vi "Demo.vi"() -> ()   [LabVIEW 2021, in "Autocomplete popup.lvlib"]
uses:
  Autocomplete popup.lvlib
  subvis/input options.ctl
  <vilib>/Utility/miscctls.llb/LVPointTypeDef.ctl
panel:
  out "Accept?":bool
  out "String":string
  in  "OK Button":bool
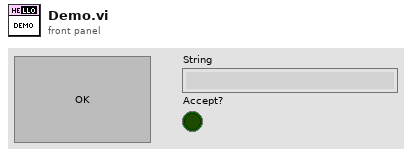
[diagram p1: front panel]
types:
  T1 = typedef "Autocomplete popup.lvlib/input options.ctl" = cluster{"Screen Coordinates":T2, "Width":u32, "max rows":i32, "List":string[], "init value":string}
  T2 = typedef "LVPointTypeDef.ctl" = cluster{"Horizontal":i16, "Vertical":i16}
  T3 = typedef "LVPositionTypeDef.ctl" = cluster{"Left":i32, "Top":i32}
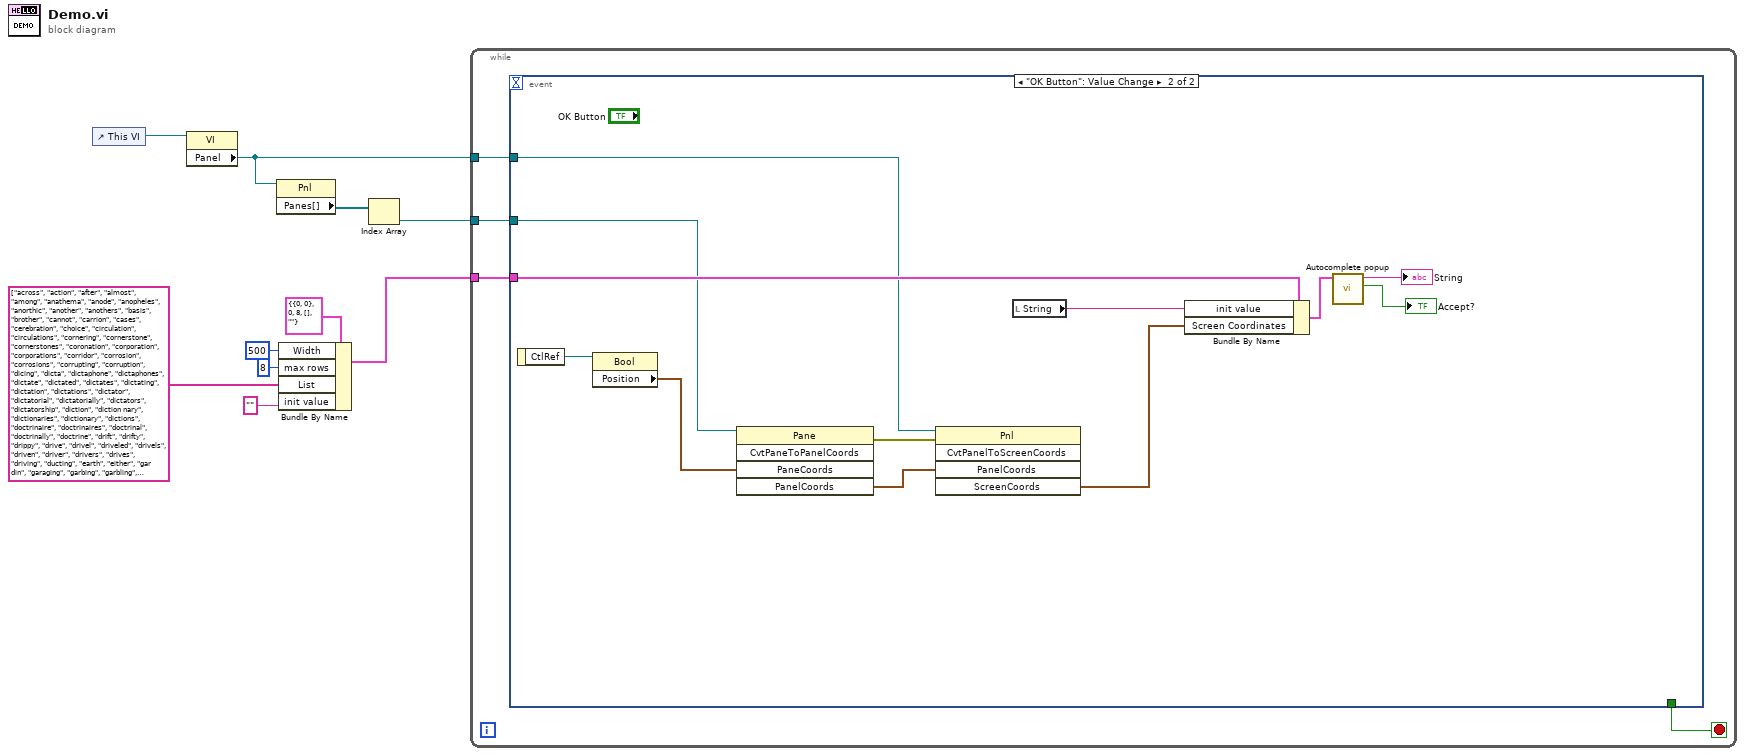
[diagram p0: block diagram]
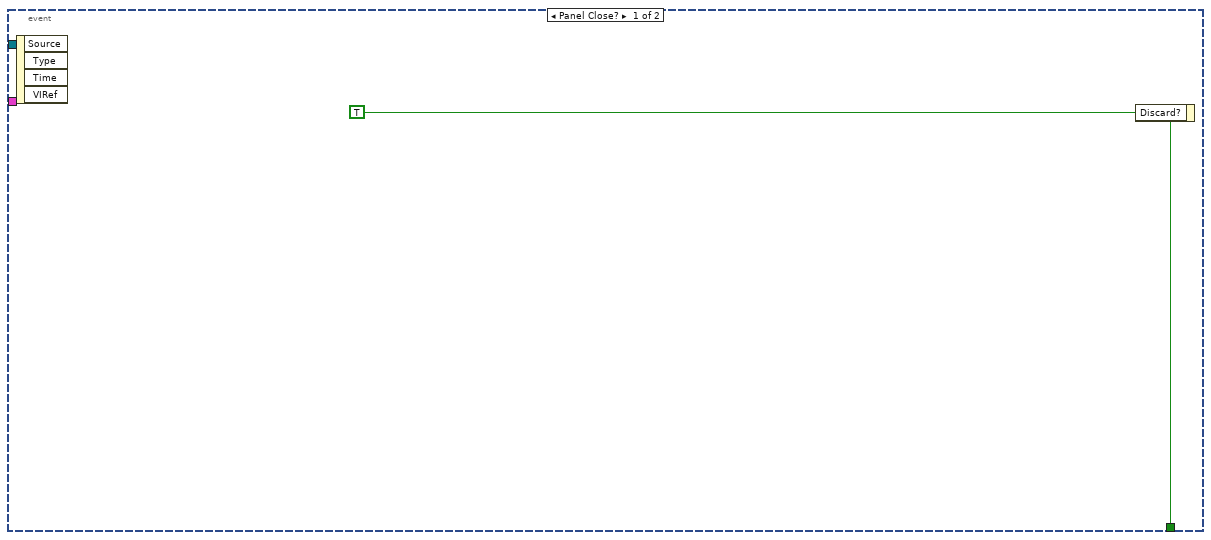
[diagram p2: hidden frame]
diagram:
  n1 = control-ref of="This VI"() -> (w5:refnum<vi>)
  n2 = property class="VI"(reference=w5) -> ("Panel"=w4:refnum<vi>)  [unwired: 1 in, 2 out]
  n3 = property class="Pnl"(reference=w4) -> ("Panes[]"=w3:refnum<vi>[])  [unwired: 1 in, 2 out]
  n4 = Bundle By Name(cluster=T1 {"Screen Coordinates"={"Horizontal"=0, "Vertical"=0}, "Width"=0, "max rows"=8, "List"=[], "init value"=""} ("input"), "Width"=u32 500, "max rows"=8, "List"=string[] ["across", "action", "after", "almost", "among", "anathema", "anode", "anopheles", "anorthic", "another", "anothers", "basis", "brother", "cannot", "carrion", "cases", "cerebration", "choice", "circulation", "circulations", "cornering", "cornerstone", "cornerstones", "coronation", "corporation", "corporations", "corridor", "corrosion", "corrosions", "corrupting", "corruption", "dicing", "dicta", "dictaphone", "dictaphones", "dictate", "dictated", "dictates", "dictating", "dictation", "dictations", "dictator", "dictatorial", "dictatorially", "dictators", "dictatorship", "diction", "diction nary", "dictionaries", "dictionary", "dictions", "doctrinaire", "doctrinaires", "doctrinal", "doctrinally", "doctrine", "drift", "drifty", "drippy", "drive", "drivel", "driveled", "drivels", "driven", "driver", "drivers", "drives", "driving", "ducting", "earth", "either", "gar din", "garaging", "garbing", "garbling", "garcon", "garde", "garden", "gardened", "gardener", "gardenia", "gardens", "gardner", "gargling", "goring", "habeas", "habited", "habits", "hebetate", "helicon", "helicopter", "helicopters", "heliotrope", "heliotropes", "heliotropism", "heliport", "hellcat", "hellcats", "hello", "helot", "helotries", "helotry", "helots", "hobbies", "hobbit", "hobbits", "hobblers", "hobbles", "hobbs", "hoboes", "hobos", "holdover", "hothead", "hotline", "hotlines", "hotpoint", "jasmine", "jasmines", "jason", "jaspers", "jests", "km art", "lateen", "lateens", "later", "lateral", "laterals", "lathe", "lather", "lathered", "latherer", "lathers", "lathery", "latter", "latterday", "latterly", "lattices", "leg ht", "legate", "legated", "legatee", "legates", "legato", "legator", "legatos", "leggett", "leghorn", "legit", "letter", "letters", "letterset", "lettersets", "liege", "lieges", "light", "likely", "lines", "lionize", "looking", "lottos", "machete", "machetes", "machine", "machined", "machines", "machinist", "machinists", "mahjong", "mahjongg", "mahoganies", "mahogany", "mahout", "mahouts", "majolica", "major", "majordomo", "majordomos", "majored", "majorette", "majorettes", "majoring", "majorities", "majority", "majors", "manta", "march", "massif", "mastic", "matador", "matadors", "matrimonial", "matrimonially", "matter", "matters", "matzo", "meant", "meccano", "mechanic", "mechanical", "mechanics", "mechanism", "mechanisms", "mechanist", "mechanistic", "mechanistically", "mechanists", "mechanize", "mechanized", "mechanizes", "meteor", "meter", "micas", "micatin", "michael", "michel", "michele", "michelin", "michelle", "michigan", "mickey", "microbic", "micron", "micronuclei", "microsoft", "might", "mighty", "mikes", "million", "mints", "minty", "mocha", "mochas", "mohair", "mohican", "mojave", "monday", "money", "monitor", "monster", "montage", "montana", "monte", "month", "monthly", "months", "monty", "mosaic", "mosaics", "moses", "mossback", "mossier", "mossiest", "mossing", "mosslike", "mossy", "mosts", "mother", "muses", "music", "musical", "musicale", "musicales", "musically", "musicals", "musician", "musicians", "mussily", "mussing", "mussy", "musts", "na iv", "na too", "naiad", "naifs", "nails", "naive", "naively", "naiveness", "naives", "naivete", "naivetes", "naivety", "natatorium", "nation", "national", "nationalism", "nationalist", "nationalistic", "nationalists", "nationalities", "nationality", "nationalize", "nationalizing", "nationally", "nationals", "nations", "neither", "nether", "nether land", "netherlander", "netherlanders", "netherlands", "netherworld", "netherworlds", "netter", "newark", "newborn", "newborns", "newer", "newly", "newmarket", "newport", "newsier", "newsy", "newton", "nicene", "niche", "niched", "niches", "niching", "nicknack", "nicknacks", "night", "nikes", "nikon", "nikons", "nohow", "notepad", "notes", "nothing", "notional", "noway", "palpitation", "palpitations", "parts", "person", "persons", "police", "policed", "polices", "policies", "policy", "poling", "polio", "polish", "polite", "politer", "politest", "politic", "politician", "politicians", "politicizing", "politick", "politicking", "politico", "politicos", "politics", "polities", "polity", "quickly", "reason", "reasons", "right", "rights", "sanative", "schedule", "scheduled", "scheduler", "schedulers", "schedules", "scheduling", "schema", "scheme", "scherzi", "scherzo", "schlep", "schlock", "schneider", "schnook", "schnooks", "scholar", "scholars", "scholl", "school", "schooled", "schooler", "schools", "schooner", "section", "semester", "semite", "senate", "senates", "senator", "senna", "sensate", "sentence", "sentenced", "sentences", "sentries", "she'd", "short", "sight", "situation", "sonant", "stuff", "swaged", "swayed", "swede", "swede en", "sweden", "swedes", "sweeper", "sweet", "sweeten", "sweetened", "sweetener", "sweeteners", "sweetening", "sweetens", "sweeter", "sweetie", "system", "systematic", "systematical", "systematics", "systematize", "systemic", "systemics", "systemize", "systemized", "systemizes", "systemizing", "systemless", "systems", "taurine", "taurines", "tautest", "technical", "touchiest", "toughest", "toughies", "touraine", "toured", "tourism", "tourist", "touristic", "touristically", "tourists", "tourneys", "until", "wander", "wanders", "wiggle", "wiggly", "wight", "wights", "winder", "winders", "windier", "winterkill", "wonder", "wonder full", "wondered", "wonderer", "wonderful", "wonderfully", "wonderfulness", "wonders", "wondrously"] ("words"), "init value"="") -> (w7:T1)
  n5 = Index Array(array=w3) -> (element=w2:refnum<vi>)  [unwired: 1 in]
  n6 = while {
    tunnel: w7 -> [w13]
    tunnel: w4 -> [w12]
    tunnel: w2 -> [w11]
    stop <- w14 stop-if-true
    n7 = event shown="[1] \"OK Button\": Value Change" {
      selector: _ -> [_ _]
      dyn-events: _ -> [_ _]
      timeout: _ -> [_ _]
      tunnel: [w15 _] -> w14
      tunnel: w13 -> [_ w25]
      tunnel: w12 -> [_ w20]
      tunnel: w11 -> [_ w19]
      event Panel Close? {
        w15 = TRUE ("Discard?")
        n8 = event-data() -> ()  [unwired: 1 in, 4 out]
        n9 = event-data("Discard?"=w15) -> ()  [unwired: 1 in, 1 out]
      }
      event "OK Button": Value Change {
        n10 = event-data() -> ("CtlRef"=w18:refnum<vi>)  [unwired: 1 in]
        n11 = property class="Bool"(reference=w18) -> ("Position"=w17:T3)  [unwired: 1 in, 2 out]
        n12 = invoke class="Pane" method="CvtPaneToPanelCoords"(reference=w19, "PaneCoords"=w17) -> (error out=w22:errorcluster, "PanelCoords"=w21:T2)  [unwired: 3 in, 3 out]
        n13 = invoke class="Pnl" method="CvtPanelToScreenCoords"(reference=w20, error in=w22, "PanelCoords"=w21) -> ("ScreenCoords"=w16:T2)  [unwired: 2 in, 4 out]
        n14 = local read "String"() -> (w24:string)
        n15 = Bundle By Name(cluster=w25, "init value"=w24, "Screen Coordinates"=w16) -> (w23:T1)
        n16 = call "Autocomplete popup.vi"("input"=w23) -> ("Accept?"=→"Accept?":bool, "String"=→"String":string)  [unwired: 8 in, 1 out]
      }
    }
  }
